vi "decodex_22.vi"() -> ()   [LabVIEW 2021]
doc: "This is a Decodex v2.1\n\nAndré Romero - 2026\nandretec@ifsc.usp.br\nIFSC - USP"
uses:
  <vilib>/Analysis/baseanly.llb/Mean (DBL).vi
  Thorlabs-Vector-Move/aptTec/Thorlabs-V2/Global Motors.vi
  <vilib>/Analysis/NI_AALBase.lvlib
panel:
  in  "Input File (.gcode)":path=path "C:/user-Lab/AndreTec/SolidWorks/blocos_3x3x3_LH_2um_LW_1um_H.gcode"
  out "Layer":dbl[][](array[numeric])=[[2.703, -53.721, 0.0, 5.0], [17.593, -36.268, 0.0, 20.0], [16.94, -34.885, 0.0, 20.0], [16.928, -26.538, 0.0, 20.0], [17.593, -26.538, 0.0, 20.0], [17.593, -26.538, 1.0, 45.0], [37.593, -26.538, 1.0, 35.0], [37.593, -25.538, 0.0, 85.0], [17.593, -25.538, 1.0, 35.0], [17.593, -24.538, 0.0, 85.0], [37.593, -24.538, 1.0, 35.0], [37.593, -23.538, 0.0, 85.0], [17.593, -23.538, 1.0, 35.0], [17.593, -22.538, 0.0, 85.0], [37.593, -22.538, 1.0, 35.0], [37.593, -22.538, 0.0, 45.0], [38.246, -22.191, 0.0, 85.0], [55.246, -22.191, 0.0, 85.0], [55.246, -0.885, 0.0, 85.0], [33.94, -0.885, 0.0, 85.0], [33.94, -17.885, 0.0, 85.0], [34.593, -18.538, 0.0, 85.0], [34.593, -18.538, 1.0, 45.0], [54.593, -18.538, 1.0, 35.0], [54.593, -17.538, 0.0, 85.0], [34.593, -17.538, 1.0, 35.0], [34.593, -16.538, 0.0, 85.0], [54.593, -16.538, 1.0, 35.0], [54.593, -15.538, 0.0, 85.0], [34.593, -15.538, 1.0, 35.0], [34.593, -14.538, 0.0, 85.0], [54.593, -14.538, 1.0, 35.0], [54.593, -13.538, 0.0, 85.0], [34.593, -13.538, 1.0, 35.0], [34.593, -12.538, 0.0, 85.0], [54.593, -12.538, 1.0, 35.0], [54.593, -11.538, 0.0, 85.0], [34.593, -11.538, 1.0, 35.0], [34.593, -10.538, 0.0, 85.0], [54.593, -10.538, 1.0, 35.0], [54.593, -9.538, 0.0, 85.0], [34.593, -9.538, 1.0, 35.0], [34.593, -8.538, 0.0, 85.0], [54.593, -8.538, 1.0, 35.0], [54.593, -7.538, 0.0, 85.0], [34.593, -7.538, 1.0, 35.0], [34.593, -6.538, 0.0, 85.0], [54.593, -6.538, 1.0, 35.0], [54.593, -5.538, 0.0, 85.0], [34.593, -5.538, 1.0, 35.0], [34.593, -4.538, 0.0, 85.0], [54.593, -4.538, 1.0, 35.0], [54.593, -3.538, 0.0, 85.0], [34.593, -3.538, 1.0, 35.0], [34.593, -2.538, 0.0, 85.0], [54.593, -2.538, 1.0, 35.0], [54.593, -2.538, 0.0, 45.0], [55.258, -2.538, 0.0, 85.0], [55.258, -19.538, 0.0, 85.0], [54.593, -19.538, 0.0, 85.0], [54.593, -19.538, 1.0, 45.0], [0.593, -19.538, 1.0, 35.0], [0.593, -18.538, 0.0, 85.0], [20.593, -18.538, 1.0, 35.0], [20.593, -17.538, 0.0, 85.0], [0.593, -17.538, 1.0, 35.0], [0.593, -16.538, 0.0, 85.0], [20.593, -16.538, 1.0, 35.0], [20.593, -15.538, 0.0, 85.0], [0.593, -15.538, 1.0, 35.0], [0.593, -14.538, 0.0, 85.0], [20.593, -14.538, 1.0, 35.0], [20.593, -13.538, 0.0, 85.0], [0.593, -13.538, 1.0, 35.0], [0.593, -12.538, 0.0, 85.0], [20.593, -12.538, 1.0, 35.0], [20.593, -11.538, 0.0, 85.0], [0.593, -11.538, 1.0, 35.0], [0.593, -10.538, 0.0, 85.0], [20.593, -10.538, 1.0, 35.0], [20.593, -9.538, 0.0, 85.0], [0.593, -9.538, 1.0, 35.0], [0.593, -8.538, 0.0, 85.0], [20.593, -8.538, 1.0, 35.0], [20.593, -7.538, 0.0, 85.0], [0.593, -7.538, 1.0, 35.0], [0.593, -6.538, 0.0, 85.0], [20.593, -6.538, 1.0, 35.0], [20.593, -5.538, 0.0, 85.0], [0.593, -5.538, 1.0, 35.0], [0.593, -4.538, 0.0, 85.0], [20.593, -4.538, 1.0, 35.0], [20.593, -3.538, 0.0, 85.0], [0.593, -3.538, 1.0, 35.0], [0.593, -2.538, 0.0, 85.0], [20.593, -2.538, 1.0, 35.0], [20.593, -2.538, 0.0, 45.0], [21.258, -2.538, 0.0, 85.0], [21.246, -0.885, 0.0, 85.0], [-0.06, -0.885, 0.0, 85.0], [-0.06, -22.191, 0.0, 85.0], [16.928, -27.538, 0.0, 85.0], [17.593, -27.538, 0.0, 85.0], [17.593, -27.538, 1.0, 45.0], [37.593, -27.538, 1.0, 35.0], [37.593, -28.538, 0.0, 85.0], [17.593, -28.538, 1.0, 35.0], [17.593, -29.538, 0.0, 85.0], [37.593, -29.538, 1.0, 35.0], [37.593, -30.538, 0.0, 85.0], [17.593, -30.538, 1.0, 35.0], [17.593, -31.538, 0.0, 85.0], [37.593, -31.538, 1.0, 35.0], [37.593, -32.538, 0.0, 85.0], [17.593, -32.538, 1.0, 35.0], [17.593, -33.538, 0.0, 85.0], [37.593, -33.538, 1.0, 35.0], [37.593, -34.538, 0.0, 85.0], [17.593, -34.538, 1.0, 35.0], [17.593, -35.538, 0.0, 85.0], [37.593, -35.538, 1.0, 35.0], [37.593, -35.538, 0.0, 45.0], [38.246, -34.885, 0.0, 85.0], [55.246, -34.885, 0.0, 85.0], [55.246, -56.191, 0.0, 85.0], [33.94, -56.191, 0.0, 85.0], [33.94, -39.191, 0.0, 85.0], [34.593, -39.538, 0.0, 85.0], [34.593, -39.538, 1.0, 45.0], [54.593, -39.538, 1.0, 35.0], [54.593, -38.538, 0.0, 85.0], [0.593, -38.538, 1.0, 35.0], [0.593, -37.538, 0.0, 85.0], [54.593, -37.538, 1.0, 35.0], [54.593, -36.538, 0.0, 85.0], [0.593, -36.538, 1.0, 35.0], [0.593, -36.538, 0.0, 45.0], [-0.072, -36.538, 0.0, 85.0], [-0.072, -39.538, 0.0, 85.0], [0.593, -39.538, 0.0, 85.0], [0.593, -39.538, 1.0, 45.0], [20.593, -39.538, 1.0, 35.0], [20.593, -40.538, 0.0, 85.0], [0.593, -40.538, 1.0, 35.0], [0.593, -41.538, 0.0, 85.0], [20.593, -41.538, 1.0, 35.0], [20.593, -42.538, 0.0, 85.0], [0.593, -42.538, 1.0, 35.0], [0.593, -43.538, 0.0, 85.0], [20.593, -43.538, 1.0, 35.0], [20.593, -44.538, 0.0, 85.0], [0.593, -44.538, 1.0, 35.0], [0.593, -45.538, 0.0, 85.0], [20.593, -45.538, 1.0, 35.0], [20.593, -46.538, 0.0, 85.0], [0.593, -46.538, 1.0, 35.0], [0.593, -47.538, 0.0, 85.0], [20.593, -47.538, 1.0, 35.0], [20.593, -48.538, 0.0, 85.0], [0.593, -48.538, 1.0, 35.0], [0.593, -49.538, 0.0, 85.0], [20.593, -49.538, 1.0, 35.0], [20.593, -50.538, 0.0, 85.0], [0.593, -50.538, 1.0, 35.0], [0.593, -51.538, 0.0, 85.0], [20.593, -51.538, 1.0, 35.0], [20.593, -52.538, 0.0, 85.0], [0.593, -52.538, 1.0, 35.0], [0.593, -53.538, 0.0, 85.0], [20.593, -53.538, 1.0, 35.0], [20.593, -54.538, 0.0, 85.0], [0.593, -54.538, 1.0, 35.0], [0.593, -54.538, 0.0, 45.0], [-0.072, -54.538, 0.0, 85.0], [-0.06, -34.885, 0.0, 85.0], [0.593, -22.203, 0.0, 85.0], [0.593, -21.538, 0.0, 85.0], [0.593, -21.538, 1.0, 45.0], [54.593, -21.538, 1.0, 35.0], [54.593, -20.538, 0.0, 85.0], [0.593, -20.538, 1.0, 35.0], [0.593, -20.538, 0.0, 45.0], [-0.072, -20.538, 0.0, 85.0], [-0.06, -56.191, 0.0, 85.0], [21.246, -56.191, 0.0, 85.0], [33.928, -40.538, 0.0, 85.0], [34.593, -40.538, 0.0, 85.0], [34.593, -40.538, 1.0, 45.0], [54.593, -40.538, 1.0, 35.0], [54.593, -41.538, 0.0, 85.0], [34.593, -41.538, 1.0, 35.0], [34.593, -42.538, 0.0, 85.0], [54.593, -42.538, 1.0, 35.0], [54.593, -43.538, 0.0, 85.0], [34.593, -43.538, 1.0, 35.0], [34.593, -44.538, 0.0, 85.0], [54.593, -44.538, 1.0, 35.0], [54.593, -45.538, 0.0, 85.0], [34.593, -45.538, 1.0, 35.0], [34.593, -46.538, 0.0, 85.0], [54.593, -46.538, 1.0, 35.0], [54.593, -47.538, 0.0, 85.0], [34.593, -47.538, 1.0, 35.0], [34.593, -48.538, 0.0, 85.0], [54.593, -48.538, 1.0, 35.0], [54.593, -49.538, 0.0, 85.0], [34.593, -49.538, 1.0, 35.0], [34.593, -50.538, 0.0, 85.0], [54.593, -50.538, 1.0, 35.0], [54.593, -51.538, 0.0, 85.0], [34.593, -51.538, 1.0, 35.0], [34.593, -52.538, 0.0, 85.0], [54.593, -52.538, 1.0, 35.0], [54.593, -53.538, 0.0, 85.0], [34.593, -53.538, 1.0, 35.0], [34.593, -54.538, 0.0, 85.0], [54.593, -54.538, 1.0, 35.0], [52.483, -53.721, 0.0, 85.0], [52.483, -53.721, 0.0, 45.0]]
  out "Motor Y":bool=TRUE
  out "Motor X":bool=TRUE
  out "Motor Z":bool=TRUE
  out "Estimated Finish Time":string="3:19:40"
  out "Total Estimated Time":string="0:06:40"
  out "Total Layer Time":string="0:00:13"
  in  "Automatic / Manual":bool=TRUE
  in  "Velocity Multiplier":dbl=1.0
  out "Current Velocity (mm/s)":dbl=20.0
  out "End Time":string="3:13 PM"
  out "Start Time":string="3:13 PM"
  out "Total Time":string="0:00:17"
  in  "Stop Button":bool
  out "Total Lines":i32=219
  out "Total Layers":i32=31
  out "Initial Z Position":dbl=-5.105264663696289 format="%#_5g"
  in  "Z Axis on/off":bool=TRUE
  in  "Layer Height (mm)":dbl=1.0
  out "Current Layer":i32=1
  out "Current Line":i32=2
  in  "Velocity (mm/s)":dbl=30.0
  in  "X":refnum<k7>(container)
  in  "Y":refnum<k7>(container)
  in  "Z":refnum<k7>(container)
  # "mm"
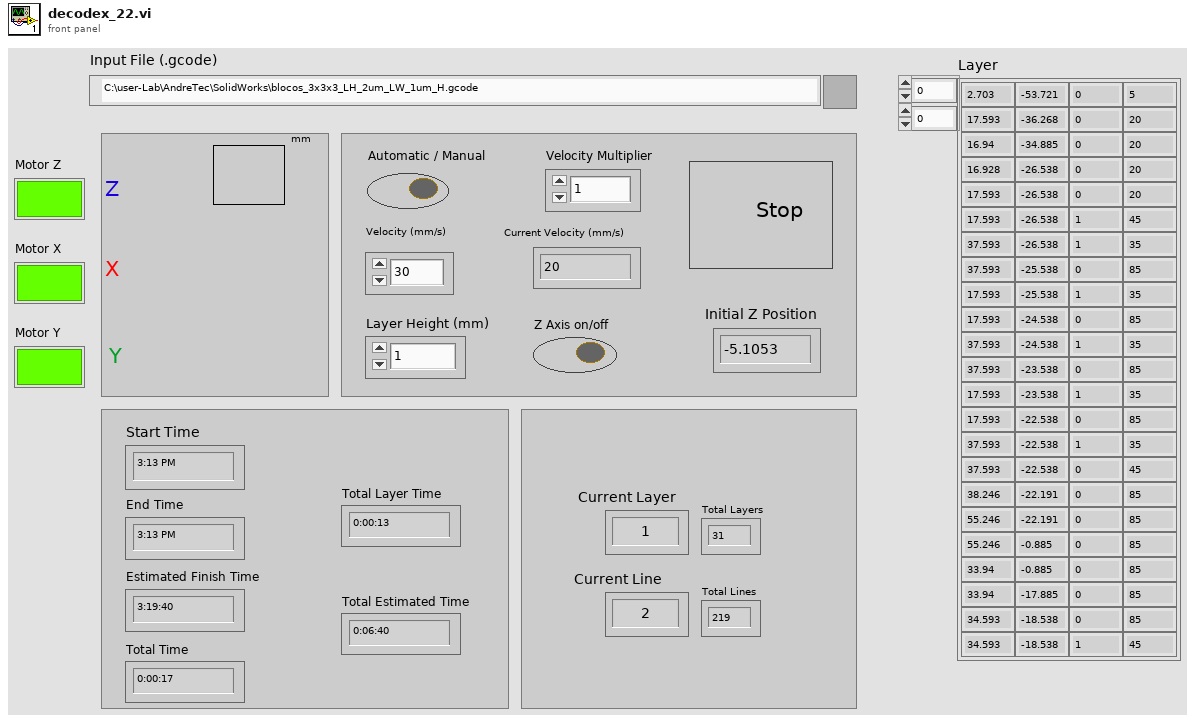
[diagram p1: front panel]
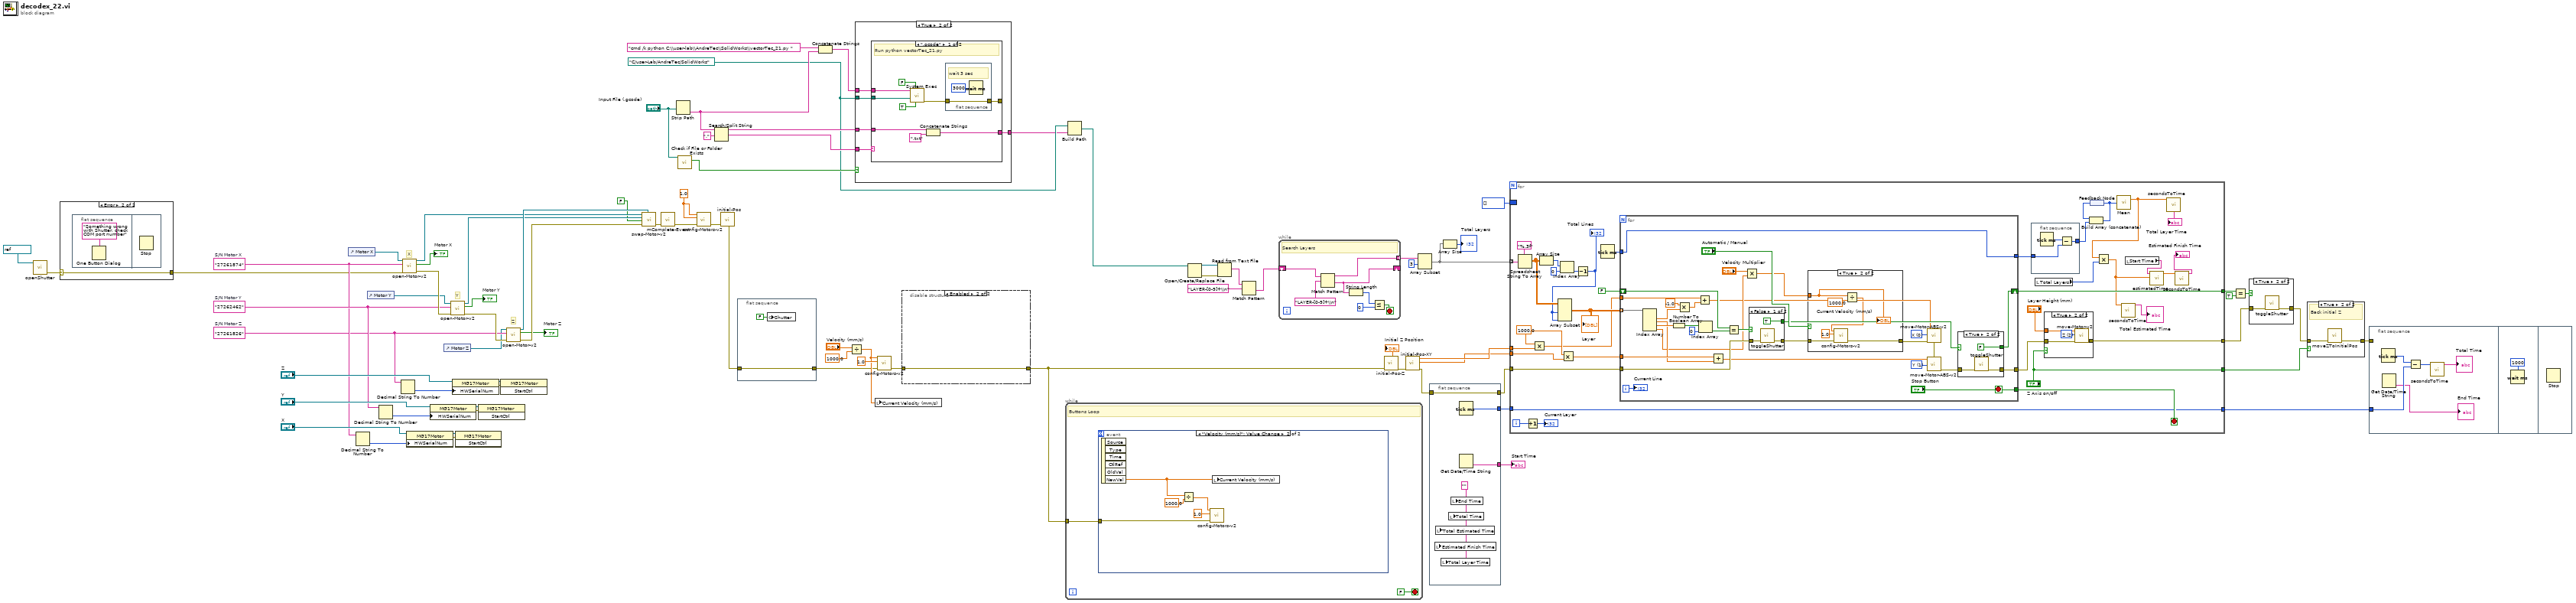
[diagram p0: block diagram]
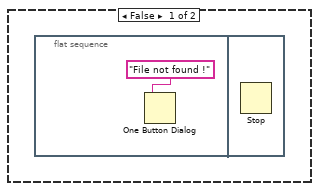
[diagram p2: hidden frame]
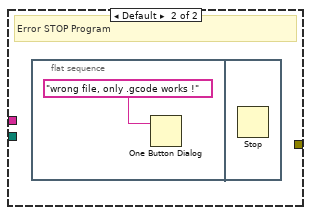
[diagram p3: hidden frame]
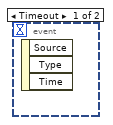
[diagram p4: hidden frame]
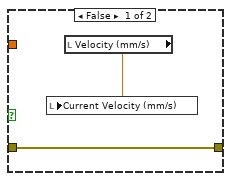
[diagram p9: hidden frame]
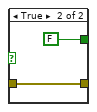
[diagram p10: hidden frame]
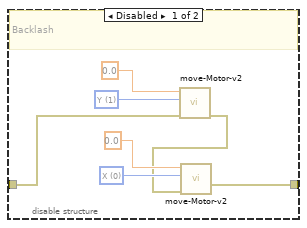
[diagram p11: hidden frame]
diagram:
  w3 = path "C:/user-Lab/AndreTec/SolidWorks" ("working directory")
  w75 = 1.0 ("Acc")
  w62 = "27262462"  # S/N Motor Y
  w61 = "27261874"  # S/N Motor X
  w52 = "27261826"  # S/N Motor Z
  # "X"
  # "Y"
  # "Z"
  n1 = call "openShutter.vi"("VISA Refnum in"=refnum<visa-resource-name> "COM3") -> ("error out"=w54:errorcluster)  [unwired: 9 in, 1 out]
  n2 = case shown="Error" w54 {
    selector: w54 -> [w81 w82]
    tunnel: [w81 w82] -> w53
    frame No Error {
    }
    frame Error {
      n3 = flat-sequence {
        frame #0 {
          n4 = One Button Dialog(message="Something wrong with Shutter, check COM port number") -> ()  [unwired: 1 in, 1 out]
        }
        frame #1 {
          n5 = Stop() -> ()  [unwired: 1 in]
        }
      }
    }
  }
  n6 = control-ref of="Motor X"() -> (w14:refnum<vi>)
  n7 = Decimal String To Number(string=w61) -> (number=w63:i32)  [unwired: 2 in, 1 out]
  n8 = control-ref of="Motor Y"() -> (w13:refnum<vi>)
  n9 = Decimal String To Number(string=w62) -> (number=w67:i32)  [unwired: 2 in, 1 out]
  n10 = Decimal String To Number(string=w52) -> (number=w71:i32)  [unwired: 2 in, 1 out]
  n11 = call "open-Motor-v2.vi"("Error In"=w53, "S/N Motor"=w61, "ref Boolean in"=w14) -> ("Error Out"=w80:errorcluster, "Motor Status"=→"Motor X":bool, "Refnum out"=w58:refnum<k7>)  [unwired: 6 in]
  n12 = property class="MG17Motor"(reference="X", "HWSerialNum"=w63) -> (reference out=w64:refnum<k7>, error out=w65:errorcluster)  [unwired: 1 in]
  n13 = property class="MG17Motor"(reference="Y", "HWSerialNum"=w67) -> (reference out=w68:refnum<k7>, error out=w69:errorcluster)  [unwired: 1 in]
  n14 = control-ref of="Motor Z"() -> (w12:refnum<vi>)
  n15 = call "open-Motor-v2.vi"("Error In"=w80, "S/N Motor"=w62, "ref Boolean in"=w13) -> ("Error Out"=w78:errorcluster, "Motor Status"=→"Motor Y":bool, "Refnum out"=w57:refnum<k7>)  [unwired: 6 in]
  n16 = property class="MG17Motor"(reference="Z", "HWSerialNum"=w71) -> (reference out=w72:refnum<k7>, error out=w73:errorcluster)  [unwired: 1 in]
  n17 = invoke class="MG17Motor" method="StartCtrl"(reference=w64, error in=w65) -> ()  [unwired: 1 in, 3 out]
  n18 = invoke class="MG17Motor" method="StartCtrl"(reference=w68, error in=w69) -> ()  [unwired: 1 in, 3 out]
  n19 = invoke class="MG17Motor" method="StartCtrl"(reference=w72, error in=w73) -> ()  [unwired: 1 in, 3 out]
  n20 = call "open-Motor-v2.vi"("Error In"=w78, "S/N Motor"=w52, "ref Boolean in"=w12) -> ("Error Out"=w77:errorcluster, "Motor Status"=→"Motor Z":bool, "Refnum out"=w76:refnum<k7>)  [unwired: 6 in]
  n21 = call "swap-Motor-v2.vi"("Refnum in M3"=w76, "error in (no error)"=w77, "Swap motor"=FALSE, "Refnum in M2"=w57, "Refnum in M1"=w58) -> ("error out"=w60:errorcluster)  [unwired: 6 in]
  n22 = call "mComplete-Event.vi"("Error In"=w60) -> ("Error Out"=w59:errorcluster)  [unwired: 10 in]
  n23 = Strip Path(path="Input File (.gcode)") -> (name=w8:string)  [unwired: 1 out]
  n24 = call <vilib>:"Check if File or Folder Exists.vi"("path"="Input File (.gcode)") -> ("file or folder exists?"=w4:bool)  [unwired: 8 in, 2 out]
  n25 = call "config-Motors-v2.vi"("error in"=w59, "Acc"=w75, "Velocity"=w75) -> ("error out"=w79:errorcluster)  [unwired: 8 in]
  n26 = Search/Split String(string=w8, search string/char (-)=".") -> (substring before match=w7:string, match + rest of string=w9:string)  [unwired: 1 in, 1 out]
  n27 = call "initial-Pos.vi"("error in (no error)"=w79) -> ("error out"=w19:errorcluster)  [unwired: 10 in]
  n28 = flat-sequence {
    tunnel: [w85] -> w20
    tunnel: w19 -> [w85]
    frame #0 {
      n29 = global write "Global Motors.vi" "Shutter"(FALSE ("Shutter")) -> ()
    }
  }
  n30 = Concatenate Strings("cmd /k python C:\\user-lab\\AndreTec\\SolidWorks\\vectorTec_21.py " ("command line"), w8) -> (w11:string)
  n31 = Divide(x="Velocity (mm/s)", y=1000.0) -> (x/y=w23:dbl)
  n32 = case shown="True" w4 {
    tunnel: w11 -> [_ w91]
    tunnel: w9 -> [_ w90]
    tunnel: w7 -> [_ w89]
    tunnel: w3 -> [_ w88]
    tunnel: [_ w87] -> w2
    frame False {
      n33 = flat-sequence {
        frame #0 {
          n34 = One Button Dialog(message="File not found !") -> ()  [unwired: 1 in, 1 out]
        }
        frame #1 {
          n35 = Stop() -> ()  [unwired: 1 in]
        }
      }
    }
    frame True {
      n36 = case shown="\".gcode\"" w90 {
        tunnel: w88 -> [w99 _]
        tunnel: w91 -> [w97 _]
        tunnel: w89 -> [w96 _]
        tunnel: [w94 _] -> w87
        tunnel: [w92 _] -> _
        frame ".gcode" {
          # "Run python vectorTec_21.py"
          n37 = call <vilib>:"System Exec.vi"("run minimized? (F)"=TRUE, "wait until completion? (T)"=FALSE, "working directory"=w99, "command line"=w97) -> ("error out"=w93:errorcluster)  [unwired: 4 in, 3 out]
          n38 = Concatenate Strings(w96, ".txt" ("string")) -> (w94:string)
          n39 = flat-sequence {
            tunnel: w93 -> [w102]
            tunnel: [w102] -> w92
            frame #0 {
              # "wait 3 sec"
              n40 = Wait (ms)(milliseconds to wait=u32 3000) -> ()  [unwired: 1 out]
            }
          }
        }
        frame Default {
          # "Error STOP Program"
          n41 = flat-sequence {
            frame #0 {
              n42 = One Button Dialog(message="wrong file, only .gcode works !") -> ()  [unwired: 1 in, 1 out]
            }
            frame #1 {
              n43 = Stop() -> ()  [unwired: 1 in]
            }
          }
        }
      }
    }
  }
  n44 = local write "Current Velocity (mm/s)"(w23) -> ()
  n45 = call "config-Motors-v2.vi"("error in"=w20, "Acc"=1.0, "Velocity"=w23) -> ("error out"=w49:errorcluster)  [unwired: 8 in]
  n46 = disable-structure shown="Enabled" {
    disable-tunnel: w49 -> [w106 w111]
    disable-tunnel: [w104 w111] -> w22
    frame Disabled {
      w109 = u16 1 items=["X", "Y", "Z"] ("Axis")
      w110 = u16 0 items=["X", "Y", "Z"] ("Axis")
      # "Backlash"
      n47 = call "move-Motor-v2.vi"("error in"=w106, "Axis"=w109, "Distance (um)"=0.0) -> ("error out"=w105:errorcluster)  [unwired: 8 in]
      n48 = call "move-Motor-v2.vi"("error in"=w105, "Axis"=w110, "Distance (um)"=0.0) -> ("error out"=w104:errorcluster)  [unwired: 8 in]
    }
    frame Enabled {
    }
  }
  n49 = while {
    tunnel: w22 -> [w112]
    stop <- FALSE stop-if-true
    # "Buttons Loop"
    n50 = event shown="[1] \"Velocity (mm/s)\": Value Change" {
      selector: _ -> [_ _]
      dyn-events: _ -> [_ _]
      timeout: _ -> [_ _]
      tunnel: w112 -> [_ w116]
      event Timeout {
        n51 = event-data() -> ()  [unwired: 1 in, 3 out]
      }
      event "Velocity (mm/s)": Value Change {
        n52 = event-data() -> ("NewVal"=w114:dbl)  [unwired: 1 in, 5 out]
        n53 = Divide(x=w114, y=1000.0) -> (x/y=w115:dbl)
        n54 = call "config-Motors-v2.vi"("error in"=w116, "Acc"=1.0, "Velocity"=w115) -> ()  [unwired: 8 in, 1 out]
        n55 = local write "Current Velocity (mm/s)"(w114) -> ()
      }
    }
  }
  n56 = Build Path(base path=w3, name or relative path=w2) -> (appended path=w1:path)
  n57 = Open/Create/Replace File(file path (use dialog)=w1) -> (refnum out=w47:refnum<file>, error out=w48:errorcluster)  [unwired: 5 in, 1 out]
  n58 = Read from Text File(file (use dialog)=w47, error in=w48) -> (text=w46:string)  [unwired: 2 in, 3 out]
  n59 = Match Pattern(string=w46, regular expression="LAYER-[0-9]+\\n") -> (after substring=w44:string)  [unwired: 1 in, 3 out]
  n60 = while {
    shift-right: [w122] -> _
    shift-left: w44 -> [w124]
    tunnel: [w119] -> w43 mode=indexing
    stop <- w120 stop-if-true
    # "Search Layers"
    n61 = Match Pattern(string=w124, regular expression="LAYER-[0-9]+\\n") -> (before substring=w119:string, after substring=w122:string)  [unwired: 1 in, 2 out]
    n62 = String Length(string=w122) -> (length=w123:i32)
    n63 = Less Or Equal?(x=w123, y=0) -> (x <= y?=w120:bool)
  }
  n64 = call "initial-Pos-Z.vi"("error in (no error)"=w22) -> ("error out"=w36:errorcluster, "Z position"=→"Initial Z Position":dbl)  [unwired: 9 in]
  n65 = call "initial-Pos-XY.vi"("error in (no error)"=w36) -> ("error out"=w29:errorcluster, "Y position"=w40:dbl, "X position"=w41:dbl)  [unwired: 8 in]
  n66 = Array Subset(array=w43, index=3) -> (w38:string[])  [unwired: 1 in]
  n67 = flat-sequence {
    tunnel: w29 -> [w129]
    tunnel: [w129] -> w28
    tunnel: [w128] -> w26
    tunnel: [w127] -> w25
    frame #0 {
      w126 = "" ("End time")
      n68 = local write "Estimated Finish Time"(w126) -> ()
      n69 = local write "Total Estimated Time"(w126) -> ()
      n70 = local write "Total Layer Time"(w126) -> ()
      n71 = local write "Total Time"(w126) -> ()
      n72 = local write "End Time"(w126) -> ()
      n73 = Tick Count (ms)() -> (millisecond timer value=w128:u32)
      n74 = Get Date/Time String() -> (time string=w127:string)  [unwired: 3 in, 1 out]
    }
  }
  n75 = Array Size(array=w38) -> (size(s)=→"Total Layers":i32)
  n76 = for {
    tunnel: w38 -> [w148] mode=indexing
    tunnel: w28 -> [w165]
    tunnel: w41 -> [w153]
    tunnel: w40 -> [w154]
    tunnel: [w160] -> w31
    tunnel: ["Z Axis on/off"] -> w39
    tunnel: [w146] -> w34
    tunnel: w26 -> [w143]
    tunnel: [w143] -> w21
    border: u32[] [] -> [_]
    i -> [w163]
    stop <- w144 stop-if-true
    w152 = 1000.0 ("x")
    n77 = Spreadsheet String To Array(format string="%.3f", spreadsheet string=w148) -> (array=w157:dbl[][])  [unwired: 2 in]
    n78 = Increment(x=w163) -> (x+1=→"Current Layer":i32)
    n79 = Multiply(x=w152, y=w153) -> (x*y=w151:dbl)
    n80 = Array Size(array=w157) -> (size(s)=w159:i32[])
    n81 = Index Array(array=w159, index=0) -> (element=w156:i32)
    n82 = Multiply(x=w152, y=w154) -> (x*y=w150:dbl)
    n83 = Decrement(x=w156) -> (x-1=w147:i32)
    "Total Lines" <- w147
    n84 = Array Subset(array=w157, length (row)=w147, length (col)=w147) -> (w155:dbl[][])  [unwired: 2 in]
    "Layer" <- w155
    n85 = Tick Count (ms)() -> (millisecond timer value=w142:u32)
    n86 = for {
      tunnel: w155 -> [w175] mode=indexing
      shift-right: [w179] -> w146
      shift-left: FALSE -> [w203]
      tunnel: w165 -> [w201]
      tunnel: [w180] -> w145
      tunnel: w151 -> [w196]
      tunnel: w150 -> [w195]
      tunnel: ["Stop Button"] -> w144
      tunnel: w142 -> [w177]
      tunnel: [w177] -> w141
      i -> [w198]
      stop <- "Stop Button" stop-if-true
      w199 = u16 1 items=["X", "Y", "Z"] ("Axis")
      w200 = u16 0 items=["X", "Y", "Z"] ("Axis")
      n87 = Index Array(array=w175) -> (element #1=w194:dbl, element #2=w193:dbl, element #3=w206:dbl, element #4=w186:dbl)  [unwired: 4 in]
      n88 = Number To Boolean Array(number=w206) -> (Boolean array=w205:bool[])
      n89 = Multiply(x=-1.0, y=w194) -> (x*y=w191:dbl)
      n90 = Add(x=w196, y=w191) -> (x+y=w176:dbl)
      n91 = Index Array(array=w205, index=0) -> (element=w183:bool)
      n92 = Add(x=w195, y=w193) -> (x+y=w189:dbl)
      n93 = Equal?(x=w203, y=w183) -> (x = y?=w202:bool)
      n94 = Multiply(x="Velocity Multiplier", y=w186) -> (x*y=w184:dbl)
      n95 = case shown="False" w202 {
        tunnel: w201 -> [w222 w224]
        tunnel: [w221 w224] -> w188
        tunnel: [TRUE FALSE] -> w178
        frame False {
          n96 = call "toggleShutter.vi"("Error In"=w222) -> ("error out"=w221:errorcluster)  [unwired: 9 in]
        }
        frame True {
        }
      }
      n97 = case shown="True" "Automatic / Manual" {
        tunnel: [w213 w219] -> w182
        tunnel: w188 -> [w213 w218]
        tunnel: w184 -> [_ w214]
        frame False {
          n98 = local read "Velocity (mm/s)"() -> (w212:dbl)
          n99 = local write "Current Velocity (mm/s)"(w212) -> ()
        }
        frame True {
          n100 = Divide(x=w214, y=1000.0) -> (x/y=w215:dbl)
          n101 = call "config-Motors-v2.vi"("error in"=w218, "Acc"=1.0, "Velocity"=w215) -> ("error out"=w219:errorcluster)  [unwired: 8 in]
          "Current Velocity (mm/s)" <- w214
        }
      }
      n102 = call "move-Motor-ABS-v2.vi"("error in"=w182, "Axis"=w200, "Distance (um)"=w176) -> ("error out"=w197:errorcluster)  [unwired: 8 in]
      n103 = call "move-Motor-ABS-v2.vi"("error in"=w197, "Axis"=w199, "Distance (um)"=w189) -> ("error out"=w181:errorcluster)  [unwired: 8 in]
      n104 = case shown="True" w178 {
        selector: w178 -> [w207 _]
        tunnel: w181 -> [w208 w211]
        tunnel: [w208 w210] -> w180
        tunnel: [w207 FALSE] -> w179
        frame False {
        }
        frame True {
          n105 = call "toggleShutter.vi"("Error In"=w211) -> ("error out"=w210:errorcluster)  [unwired: 9 in]
        }
      }
      "Current Line" <- w198
    }
    n106 = flat-sequence {
      tunnel: w141 -> [w168]
      tunnel: [w167] -> w139
      frame #0 {
        n107 = Tick Count (ms)() -> (millisecond timer value=w169:u32)
        n108 = Subtract(x=w169, y=w168) -> (x-y=w167:u32)
      }
    }
    n109 = local read "Total Layers"() -> (w135:i32)
    n110 = case shown="True" "Z Axis on/off" {
      tunnel: "Layer Height (mm)" -> [_ w173]
      tunnel: [w170 w172] -> w160
      tunnel: w145 -> [w170 w171]
      frame False {
      }
      frame True {
        w174 = u16 2 items=["X", "Y", "Z"] ("Axis")
        n111 = call "move-Motor-v2.vi"("error in"=w171, "Axis"=w174, "Distance (um)"=w173) -> ("error out"=w172:errorcluster)  [unwired: 8 in]
      }
    }
    n112 = feedback #1() -> (w138:u32[])
    n113 = Build Array (concatenate)(w138, w139) -> (w137:u32[])
    n114 = feedback-in #1(w137) -> ()
    n115 = call-poly <vilib>:"Mean.vi"("X"=w137) -> ("mean"=w133:dbl)  [unwired: 1 out]
    n116 = Multiply(x=w133, y=w135) -> (x*y=w130:dbl)
    n117 = call "secondsToTime.vi"("Time input (ms)"=w130) -> ("Time Stamp"=→"Total Estimated Time":string)  [unwired: 10 in]
    n118 = local read "Start Time"() -> (w134:string)
    n119 = call "estimatedTime.vi"("time (ms)"=w130, "Start time"=w134) -> ("total time"=w132:dbl)  [unwired: 9 in]
    n120 = call "secondsToTime.vi"("Time input (ms)"=w133) -> ("Time Stamp"=→"Total Layer Time":string)  [unwired: 10 in]
    n121 = call "secondsToTime.vi"("Time input (ms)"=w132) -> ("Time Stamp"=→"Estimated Finish Time":string)  [unwired: 10 in]
  }
  n122 = Equal?(x=w34, y=TRUE) -> (x = y?=w32:bool)
  n123 = case shown="True" w32 {
    tunnel: w31 -> [w225 w227]
    tunnel: [w225 w226] -> w30
    frame False {
    }
    frame True {
      n124 = call "toggleShutter.vi"("Error In"=w227) -> ("error out"=w226:errorcluster)  [unwired: 9 in]
    }
  }
  n125 = case shown="True" w39 {
    tunnel: [w228 w230] -> w27
    tunnel: w30 -> [w228 w229]
    frame False {
    }
    frame True {
      # "Back initial Z"
      n126 = call "moveZToInitialPos.vi"("error in"=w229) -> ("error out"=w230:errorcluster)  [unwired: 10 in]
    }
  }
  n127 = flat-sequence {
    tunnel: w27 -> [_]
    tunnel: w21 -> [w232]
    frame #0 {
      n128 = Tick Count (ms)() -> (millisecond timer value=w233:u32)
      n129 = Get Date/Time String() -> (time string=→"End Time":string)  [unwired: 3 in, 1 out]
      n130 = Subtract(x=w233, y=w232) -> (x-y=w234:u32)
      n131 = call "secondsToTime.vi"("Time input (ms)"=w234) -> ("Time Stamp"=→"Total Time":string)  [unwired: 10 in]
    }
    frame #1 {
      n132 = Wait (ms)(milliseconds to wait=u32 1000) -> ()  [unwired: 1 out]
    }
    frame #2 {
      n133 = Stop() -> ()  [unwired: 1 in]
    }
  }
  "Start Time" <- w25
